vi "Create Assert Factory.vi"(7 "Interactive":bool, 8 "error in (no error)":errorcluster, 9 "Test Report":refnum<class "Test Report.lvclass">, 10 "Verbose (F)":bool, 11 "Test Assert Factory in":refnum<class "Test Assert Factory.lvclass">) -> (0 "error out":errorcluster, 3 "Test Assert Factory out":refnum<class "Test Assert Factory.lvclass">)   [LabVIEW 2013, in "Caraya.lvlib" / "Test Assert Factory.lvclass"]
uses:
  Test Assert Factory.lvclass
  Test Report/Test Report.lvclass
  Test Result/Test Result.lvclass
  Test Result/Test Events -- cluster.ctl
  Test Report/Test Report.lvclass/Test Report.ctl
  Test Assert Factory.lvclass/Test Assert Factory.ctl
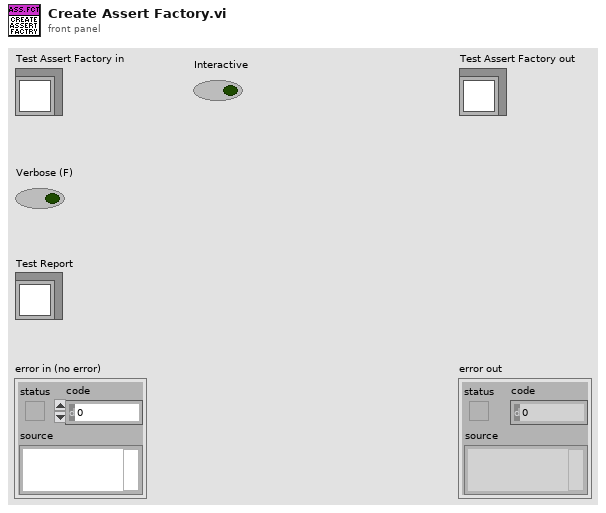
[diagram p1: front panel]
types:
  T1 = typedef "Caraya.lvlib/Test Result.lvclass/Test Events -- cluster.ctl" = cluster{"Test Registration Event":refnum<user-event>, "Assertion Event":refnum<user-event>, "Assertion Update Event":refnum<user-event>}
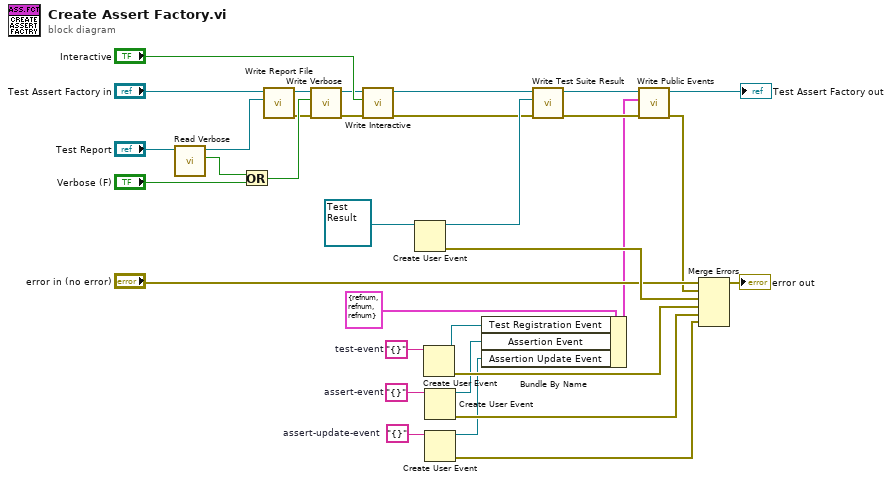
[diagram p0: block diagram]
diagram:
  w15 = "{}"  # assert-update-event
  w16 = "{}"  # assert-event
  w17 = "{}"  # test-event
  n1 = call "Read Verbose.vi"("Test Report in"="Test Report") -> ("Verbose"=w31:bool, "Test Report out"=w29:refnum<class "Test Report.lvclass">)  [unwired: 8 in, 1 out]
  n2 = Or(x=w31, y="Verbose (F)") -> (x .or. y?=w25:bool)
  n3 = call "Write Report File.vi"("Test Report"=w29, "Test Assert Factory in"="Test Assert Factory in") -> ("error out"=w24:errorcluster, "Test Assert Factory out"=w27:refnum<class "Test Assert Factory.lvclass">)  [unwired: 8 in]
  n4 = call "Write Verbose.vi"("error in (no error)"=w24, "Verbose"=w25, "Test Assert Factory in"=w27) -> ("error out"=w23:errorcluster, "Test Assert Factory out"=w26:refnum<class "Test Assert Factory.lvclass">)  [unwired: 7 in]
  n5 = call "Write Interactive.vi"("error in (no error)"=w23, "Interactive"="Interactive", "Test Assert Factory in"=w26) -> ("error out"=w1:errorcluster, "Test Assert Factory out"=w2:refnum<class "Test Assert Factory.lvclass">)  [unwired: 7 in]
  n6 = Create User Event(user event datatype=refnum<class "Test Result.lvclass"> refnum ("Test Result")) -> (user event=w18:refnum<user-event>, error out=w21:errorcluster)  [unwired: 1 in]
  n7 = Create User Event(user event datatype=w17) -> (user event=w6:refnum<user-event>, error out=w10:errorcluster)  [unwired: 1 in]
  n8 = Create User Event(user event datatype=w16) -> (user event=w5:refnum<user-event>, error out=w9:errorcluster)  [unwired: 1 in]
  n9 = Create User Event(user event datatype=w15) -> (user event=w4:refnum<user-event>, error out=w8:errorcluster)  [unwired: 1 in]
  n10 = Bundle By Name(cluster=T1 {"Test Registration Event"=refnum, "Assertion Event"=refnum, "Assertion Update Event"=refnum} ("Public Events"), "Test Registration Event"=w6, "Assertion Event"=w5, "Assertion Update Event"=w4) -> (w3:T1)
  n11 = call "Write Test Suite Result.vi"("error in (no error)"=w1, "Test Suite Result"=w18, "Test Assert Factory in"=w2) -> ("error out"=w12:errorcluster, "Test Assert Factory out"=w14:refnum<class "Test Assert Factory.lvclass">)  [unwired: 7 in]
  n12 = call "Write Public Events.vi"("error in (no error)"=w12, "Public Events"=w3, "Test Assert Factory in"=w14) -> ("error out"=w11:errorcluster, "Test Assert Factory out"=→"Test Assert Factory out":refnum<class "Test Assert Factory.lvclass">)  [unwired: 7 in]
  n13 = Merge Errors("error in (no error)", w11, w21, w10, w9, w8) -> (→"error out":errorcluster)
